vi "DateTime_OS-indep.vi"() -> (0 "Time":string, 1 "Date":string)   [LabVIEW 2013]
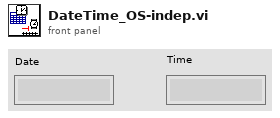
[diagram p1: front panel]
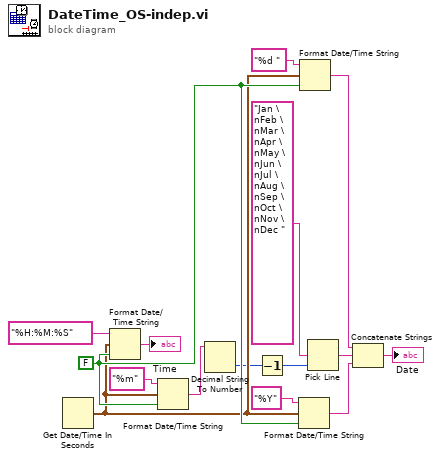
[diagram p0: block diagram]
diagram:
  w13 = FALSE
  n1 = Get Date/Time In Seconds() -> (seconds since 1Jan1904=w12:timestamp)
  n2 = Format Date/Time String(time format string (%c)="%H:%M:%S", seconds (now)=w12, UTC format=w13) -> (date/time string=→"Time":string)
  n3 = Format Date/Time String(time format string (%c)="%m", seconds (now)=w12, UTC format=w13) -> (date/time string=w8:string)
  n4 = Decimal String To Number(string=w8) -> (number=w2:i32)  [unwired: 2 in, 1 out]
  n5 = Decrement(x=w2) -> (x-1=w1:i32)
  n6 = Format Date/Time String(time format string (%c)="%Y", seconds (now)=w12, UTC format=w13) -> (date/time string=w5:string)
  n7 = Format Date/Time String(time format string (%c)="%d ", seconds (now)=w12, UTC format=w13) -> (date/time string=w6:string)
  n8 = Pick Line(multi-line string="Jan \nFeb \nMar \nApr \nMay \nJun \nJul \nAug \nSep \nOct \nNov \nDec ", line index=w1) -> (output string=w4:string)  [unwired: 1 in]
  n9 = Concatenate Strings(w6, w4, w5) -> (→"Date":string)
